vi "Send Commands(SubVI).vi"(8 "Prediction?":bool, 10 "Number of Particles after":i32, 11 "Cluster":T2) -> (0 "Predicted Position":T1, 1 "Current position":T1)   [LabVIEW 2014]
uses:
  Others/Global.vi
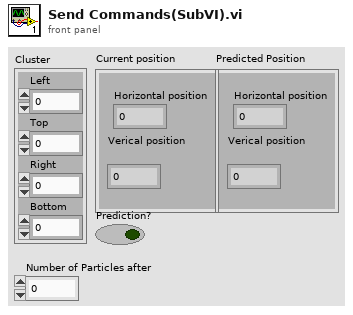
[diagram p1: front panel]
types:
  T1 = cluster{"Horizontal position":dbl, "Verical position\n":dbl}
  T2 = cluster{"Left":dbl, "Top":dbl, "Right":dbl, "Bottom":dbl}
  T3 = typedef "Control cluster.ctl" = cluster{"Roll":sgl, "Pitch":sgl, "Vertical Speed":sgl, "Yaw Speed":sgl}
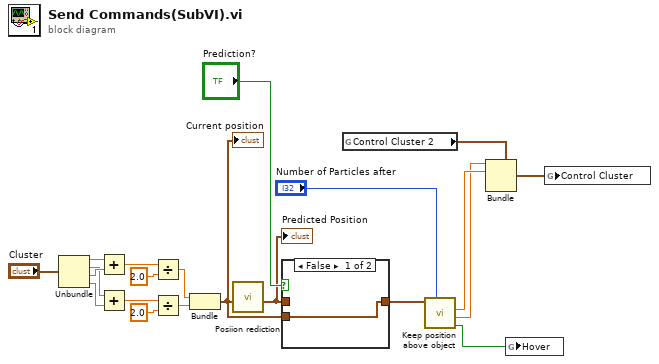
[diagram p0: block diagram]
diagram:
  n1 = Unbundle("Cluster") -> ("Left"=w14:dbl, "Top"=w3:dbl, "Right"=w4:dbl, "Bottom"=w2:dbl)
  n2 = Add(x=w14, y=w4) -> (x+y=w17:dbl)
  n3 = Add(x=w3, y=w2) -> (x+y=w18:dbl)
  n4 = Divide(x=w17, y=2.0) -> (x/y=w6:dbl)
  n5 = Divide(x=w18, y=2.0) -> (x/y=w5:dbl)
  n6 = Bundle(w6, w5) -> (w7:cluster{dbl, dbl})  [unwired: 1 in]
  "Current position" <- w7
  n7 = call "Posiion rediction.vi"("Current Position"=w7) -> ("Predicted Position"=w10:T1)  [unwired: 9 in, 1 out]
  "Predicted Position" <- w10
  n8 = case shown="False" "Prediction?" {
    tunnel: [w22 w23] -> w13
    tunnel: w10 -> [_ w23]
    tunnel: w7 -> [w22 _]
    frame False {
    }
    frame True {
    }
  }
  n9 = global read "Global.vi" "Control Cluster 2"() -> (w21:T3)
  n10 = call "Keep position above object.vi"("nr of particles"="Number of Particles after", "Position In"=w13) -> ("Hover"=w1:bool, "Roll"=w8:dbl, "Pitch"=w9:dbl)  [unwired: 6 in, 1 out]
  n11 = Bundle(cluster=w21, "Roll"=w8, "Pitch"=w9) -> (w19:T3)  [unwired: 2 in]
  n12 = global write "Global.vi" "Hover"(w1) -> ()
  n13 = global write "Global.vi" "Control Cluster"(w19) -> ()
